vi "Get Session.vi"(11 "Processing in":refnum<class "Processing.lvclass">) -> (2 "Session":refnum<class "Session.lvclass">, 3 "Processing out":refnum<class "Processing.lvclass">)   [LabVIEW 2020, in "HTTP Server.lvlib" / "Processing.lvclass"]
uses:
  Processing.lvclass
  Session/Session.lvclass
  Processing.lvclass/Processing.ctl
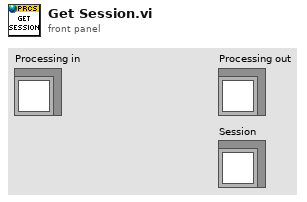
[diagram p1: front panel]
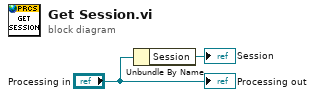
[diagram p0: block diagram]
diagram:
  n1 = Unbundle By Name("Processing in") -> ("Session"=→"Session":refnum<class "Session.lvclass">)
  "Processing out" <- "Processing in"
